vi "Get Argument.vi"(8 "error in (no error)":errorcluster, 10 "Name":string, 11 "LV Argument Parser in":refnum<class "LV Argument Parser.lvclass">) -> (0 "error out":errorcluster, 1 "key not found?":bool, 2 "element":variant, 3 "LV Argument Parser out":refnum<class "LV Argument Parser.lvclass">)   [LabVIEW 2022 SP3, in "LV ArgParse.lvlib" / "LV Argument Parser.lvclass"]
uses:
  LV Argument Parser.lvclass
  LV Argument Parser.lvclass/LV Argument Parser.ctl
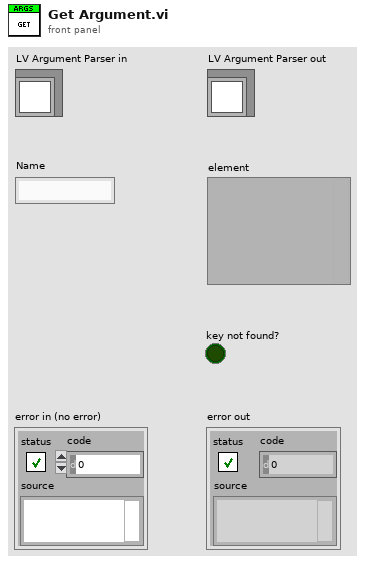
[diagram p1: front panel]
types:
  T1 = typedef "LV ArgParse.lvlib/LV Argument Parser.lvclass/Argument Definition.ctl" = cluster{"Name":string, "short (positional)":string, "long (positional)":string, "action":enum16{"store", "store-const", "store-false", "store-true", "append", "append-const", "count", "help", "version"}, "choices":string[], "const":string, "default":string, "dest (=name)":string, "help":string, "Number":i32, "Required":bool, "Type":enum16{"String", "Int", "UInt", "Float", "Bool", "Date", "Path"}}
  T2 = enum16{"store", "store-const", "store-false", "store-true", "append", "append-const", "count", "help", "version"}
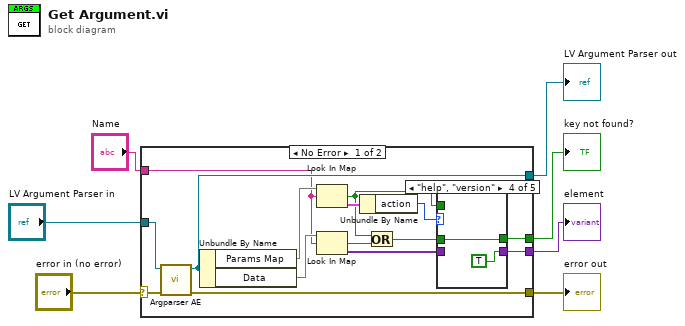
[diagram p0: block diagram]
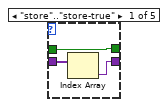
[diagram p2: hidden frame]
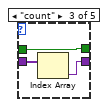
[diagram p4: hidden frame]
diagram:
  n1 = case shown="No Error" "error in (no error)" {
    selector: "error in (no error)" -> [w22 w35]
    tunnel: [w21 w35] -> w6
    tunnel: [w19 w34] -> w4
    tunnel: "LV Argument Parser in" -> [w20 w34]
    tunnel: "Name" -> [w16 _]
    tunnel: [w12 _] -> w2
    tunnel: [w9 _] -> w1
    frame No Error {
      n2 = call "Argparser AE.vi"("error in (no error)"=w22, "LV Argument Parser in"=w20) -> ("error out"=w21:errorcluster, "LV Argument Parser out"=w19:refnum<class "LV Argument Parser.lvclass">)  [unwired: 8 in]
      n3 = Unbundle By Name(w19) -> ("Params Map"=w17:map{string, T1}, "Data"=w18:map{string, variant[]})
      n4 = Look In Map(map=w17, key=w16) -> (key not found?=w10:bool, value=w15:T1)  [unwired: 1 in]
      n5 = Look In Map(map=w18, key=w16) -> (key not found?=w11:bool, value=w13:variant[])  [unwired: 1 in]
      n6 = Unbundle By Name(w15) -> ("action"=w14:T2)
      n7 = Or(x=w10, y=w11) -> (x .or. y?=w8:bool)
      n8 = case shown="\"help\", \"version\"" w14 {
        tunnel: w13 -> [w25 w27 w30 _ _]
        tunnel: [w24 w27 w29 TRUE _] -> w12
        tunnel: w10 -> [_ _ _ _ _]
        tunnel: [w23 w26 w28 w31 w33] -> w9
        tunnel: w8 -> [w23 w26 w28 w31 w33]
        frame "store".."store-true" {
          n9 = Index Array(array=w25) -> (element=w24:variant)  [unwired: 1 in]
        }
        frame "append", "append-const" {
        }
        frame "count" {
          n10 = Index Array(array=w30) -> (element=w29:variant)  [unwired: 1 in]
        }
        frame "help", "version" {
        }
        frame Default {
        }
      }
    }
    frame Error {
    }
  }
  "error out" <- w6
  "LV Argument Parser out" <- w4
  "element" <- w2
  "key not found?" <- w1
